vi "FPGA Audio Streaming.vi"() -> ()   [LabVIEW 2022 SP3]
doc: "This VI contains the default FPGA personality in addition to code that filters data based on Frequency Selector and sends data to RT Main.vi through FIFO. Keeping the default personality allows you to continue using the myRIO APIs even after adding custom FPGA code."
uses:
  <vilib>/rvi/Emulation/niFpgaGetClockAttributes.vi
  <vilib>/rvi/Emulation/niFpgaSctlEmulationGetInTimedLoop.vi
  <vilib>/rvi/Emulation/niFpgaEmulationReportErrorSimple.vi
  <vilib>/rvi/interface/RandomDataEmulation/niFpgaRandomDataHandleErrors.vi
  <vilib>/rvi/eio/common/nirviEmuTemplateMethod_errors.vi
  <vilib>/rvi/Emulation/niFpgaCriticalErrorInLSC.vi
  <vilib>/rvi/DataTransferAndStorage/Container/XNode/niFpgaContainer.xnode
  <vilib>/rvi/interface/RandomDataEmulation/nirviRandomDataFpgaReadWriteTemplate.vi
  <vilib>/eio/EIONode/EIONode.xnode
panel:
  in  "LEDs On?":bool
  in  "Count(Ticks)":u32=907
  out "Actual Period (tics)":u32
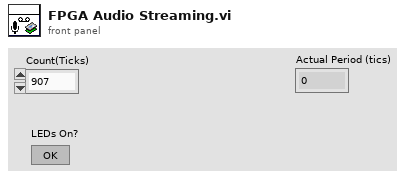
[diagram p1: front panel]
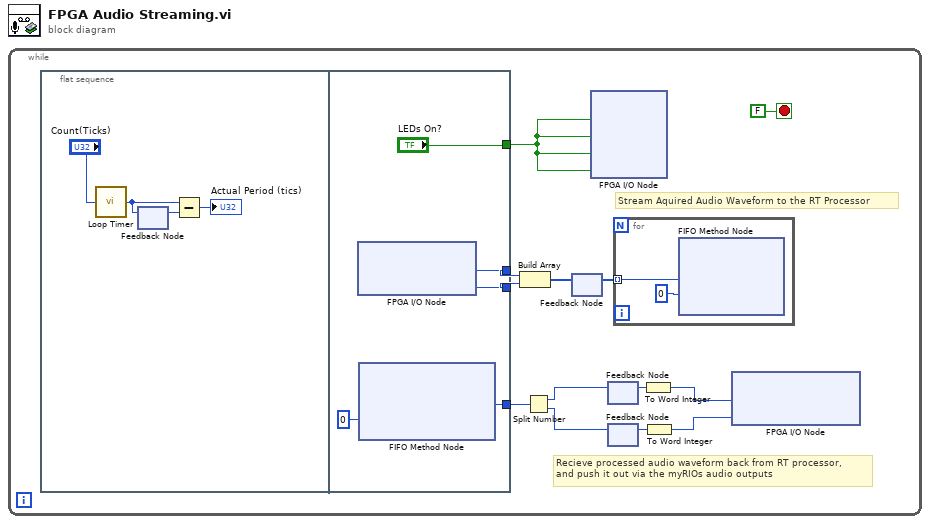
[diagram p0: block diagram]
diagram:
  n1 = while {
    stop <- FALSE stop-if-true
    # "Recieve processed audio waveform back from RT processor,\nand push it out via the myRIOs audio outputs"
    # "Stream Aquired Audio Waveform to the RT Processor"
    n2 = flat-sequence {
      tunnel: [w24] -> w10
      tunnel: [w23] -> w9
      tunnel: [w21] -> w2
      tunnel: ["LEDs On?"] -> w1
      frame #0 {
        n3 = call "Loop Timer"("Count(Ticks)"="Count(Ticks)") -> ("Tick Count(Ticks)"=w18:u32)
        n4 = feedback-in #1(w18) -> ()
        n5 = feedback #1() -> (w17:u32)  [unwired: 1 in]
        n6 = Subtract(x=w18, y=w17) -> (x-y=→"Actual Period (tics)":u32)
      }
      frame #1 {
        n7 = xnode "FPGA I/O Node"() -> ("AudioIn/Left"=w24:i16, "AudioIn/Right"=w23:i16)  [unwired: 2 in, 2 out]
        n8 = xnode ("FIFO Method Node")("Timeout"=0) -> ("Element"=w21:u32)  [unwired: 1 in, 2 out]
      }
    }
    n9 = Build Array(w10, w9) -> (w12:i16[])
    n10 = Split Number(x=w2) -> (hi(x)=w7:u16, lo(x)=w6:u16)
    n11 = feedback-in #2(w12) -> ()
    n12 = feedback #2() -> (w11:i16[])  [unwired: 1 in]
    n13 = xnode "FPGA I/O Node"("LED0"=w1, "LED1"=w1, "LED2"=w1, "LED3"=w1) -> ()  [unwired: 4 in, 4 out]
    n14 = feedback-in #3(w7) -> ()
    n15 = feedback #3() -> (w8:u16)  [unwired: 1 in]
    n16 = feedback #4() -> (w5:u16)  [unwired: 1 in]
    n17 = feedback-in #4(w6) -> ()
    n18 = for {
      tunnel: w11 -> [w15] mode=indexing
      n19 = xnode ("FIFO Method Node")("Element"=w15, "Timeout"=0) -> ()  [unwired: 1 in, 2 out]
    }
    n20 = To Word Integer(number=w8) -> (16bit integer=w3:i16)
    n21 = To Word Integer(number=w5) -> (16bit integer=w4:i16)
    n22 = xnode "FPGA I/O Node"("AudioOut/Left"=w3, "AudioOut/Right"=w4) -> ()  [unwired: 2 in, 2 out]
  }
